vi "Get Control Refnum.vi"(8 "error in (no error)":errorcluster, 11 "GUI Control in":refnum<class "GUI Control.lvclass">) -> (0 "error out":errorcluster, 2 "Ctl Refnum":refnum<vi>, 3 "GUI Control out":refnum<class "GUI Control.lvclass">)   [LabVIEW 2015, in "GUI Control.lvclass"]
uses:
  GUI Control.lvclass
  GUI Control.lvclass/GUI Control.ctl
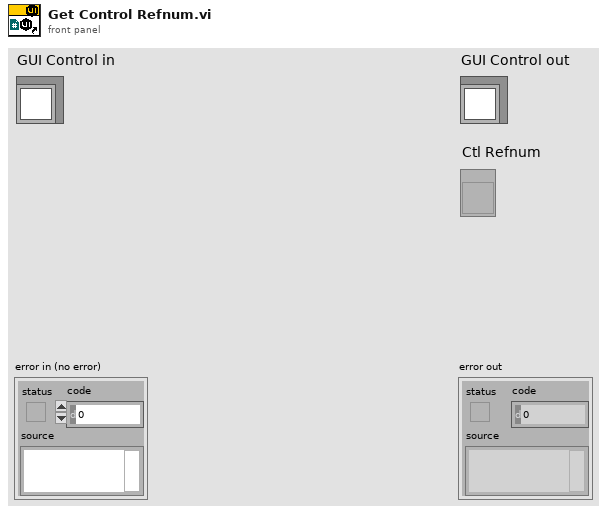
[diagram p1: front panel]
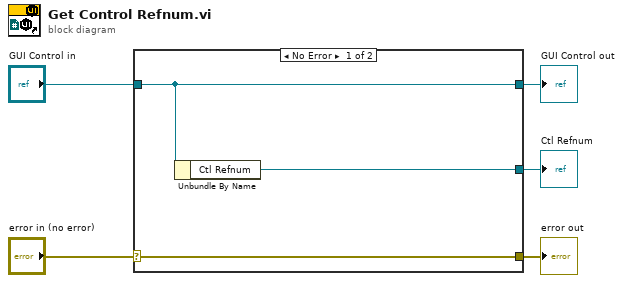
[diagram p0: block diagram]
diagram:
  n1 = case shown="No Error" "error in (no error)" {
    selector: "error in (no error)" -> [w8 w9]
    tunnel: [w8 w9] -> w4
    tunnel: [w7 w10] -> w2
    tunnel: "GUI Control in" -> [w7 w10]
    tunnel: [w6 _] -> w1
    frame No Error {
      n2 = Unbundle By Name(w7) -> ("Ctl Refnum"=w6:refnum<vi>)
    }
    frame Error {
    }
  }
  "error out" <- w4
  "GUI Control out" <- w2
  "Ctl Refnum" <- w1
